vi "Swap CASN_TRIM and HVDDL_TRIM.vi"(11 "MICS DATA INITIAL":string) -> (3 "MICS DATA FINAL":string="NaN")   [LabVIEW 2010]
panel:
  out "Trim List 2 Final Values":string[](array[string])
  out "Trim List 2 Initial Values":string[](array[string])
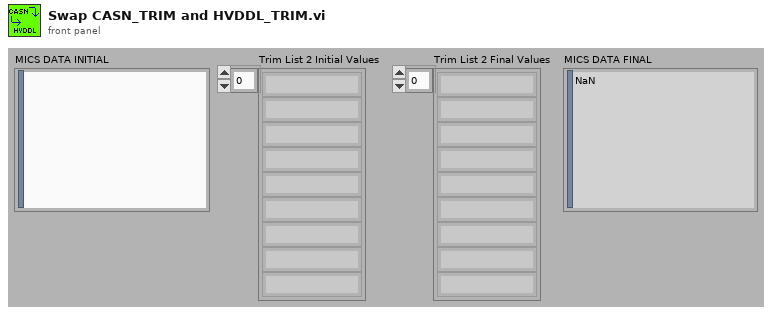
[diagram p1: front panel]
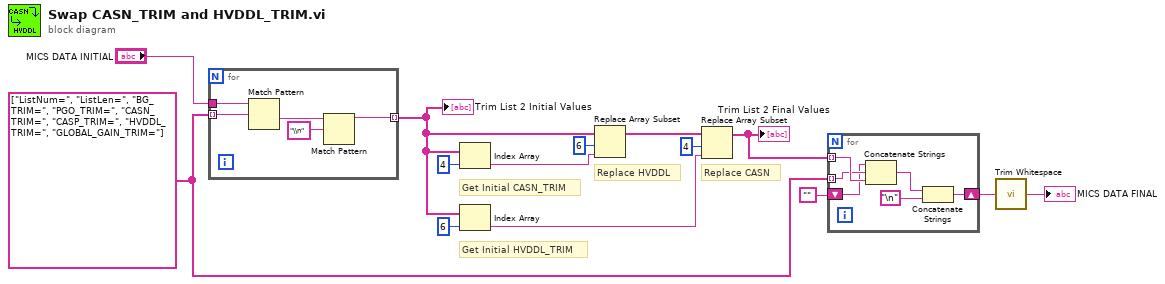
[diagram p0: block diagram]
diagram:
  w4 = string[] ["ListNum=", "ListLen=", "BG_TRIM=", "PGO_TRIM=", "CASN_TRIM=", "CASP_TRIM=", "HVDDL_TRIM=", "GLOBAL_GAIN_TRIM="]
  # "Replace CASN"
  # "Replace HVDDL"
  # "Get Initial HVDDL_TRIM"
  # "Get Initial CASN_TRIM"
  n1 = for {
    tunnel: w4 -> [w17] mode=indexing
    tunnel: [w16] -> w9 mode=indexing
    tunnel: "MICS DATA INITIAL" -> [w15]
    n2 = Match Pattern(string=w15, regular expression=w17) -> (after substring=w18:string)  [unwired: 1 in, 3 out]
    n3 = Match Pattern(string=w18, regular expression="\\n") -> (before substring=w16:string)  [unwired: 1 in, 3 out]
  }
  "Trim List 2 Initial Values" <- w9
  n4 = Index Array(array=w9, index=4) -> (element=w11:string)
  n5 = Index Array(array=w9, index=6) -> (element=w6:string)
  n6 = Replace Array Subset(array=w9, new element=w11, index=6) -> (w8:string[])
  n7 = Replace Array Subset(array=w8, new element=w6, index=4) -> (w5:string[])
  "Trim List 2 Final Values" <- w5
  n8 = for {
    tunnel: w5 -> [w22] mode=indexing
    tunnel: w4 -> [w21] mode=indexing
    shift-right: [w24] -> w1
    shift-left: "" -> [w20]
    n9 = Concatenate Strings(w20, w21, w22) -> (w25:string)
    n10 = Concatenate Strings(w25, "\n") -> (w24:string)
  }
  n11 = call <vilib>:"Trim Whitespace.vi"("string"=w1) -> ("trimmed string"=→"MICS DATA FINAL":string)  [unwired: 1 in]
